vi "Init DH20vi.vi"(8 "error in (no error)":errorcluster, 11 "Grove Temperature Humidity Sensor DH20 in":refnum<class "Grove Temperature Humidity Sensor DH20.lvclass">) -> (0 "error out":errorcluster, 3 "6Grove Temperature Humidity Sensor DH20 out":refnum<class "Grove Temperature Humidity Sensor DH20.lvclass">)   [LabVIEW 2020, in "CTI-Peripheral.lvlib" / "Grove Temperature Humidity Sensor DH20.lvclass"]
uses:
  Grove Temperature Humidity Sensor DH20.lvclass
  Grove Temperature Humidity Sensor DH20.lvclass/Grove Temperature Humidity Sensor DH20.ctl
  CTI/I2C Connection/I2C Connection.lvclass/I2C Connection.ctl
  CTI/Session/I2C Write Data.vi
  CTI/Session/I2C Read Data.vi
  CTI/I2C Connection/I2C Connection.lvclass
panel:
  out "TimedOut":bool
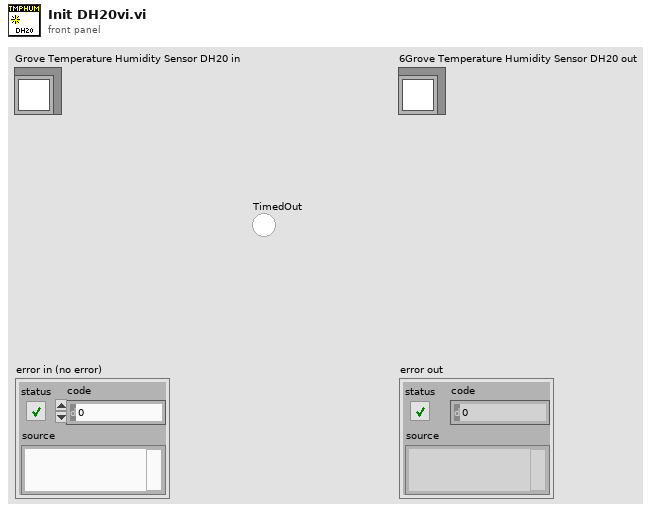
[diagram p1: front panel]
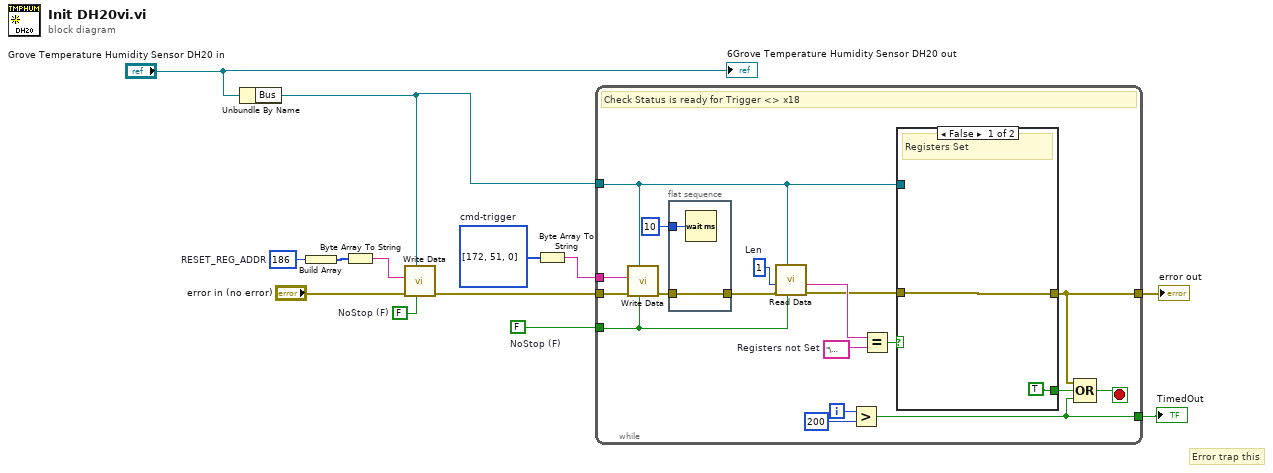
[diagram p0: block diagram]
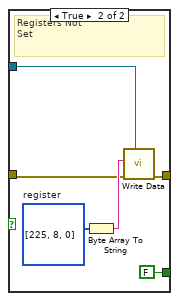
[diagram p2: hidden frame]
diagram:
  w2 = FALSE  # NoStop (F)
  w7 = FALSE  # NoStop (F)
  w9 = u8[] [172, 51, 0]  # cmd-trigger
  w12 = u8 186  # RESET_REG_ADDR
  # "Error trap this"
  n1 = Unbundle By Name("Grove Temperature Humidity Sensor DH20 in") -> ("Bus"=w3:refnum<class "I2C Connection.lvclass">)
  n2 = Build Array(w12) -> (w11:u8[])
  n3 = Byte Array To String(unsigned byte array=w11) -> (string=w6:string)
  n4 = call "Write Data.vi"("NoStop (F)"=w7, "I2C Connection"=w3, "error in (no error)"="error in (no error)", "Data"=w6) -> ("error out"=w4:errorcluster)  [unwired: 7 in]
  n5 = Byte Array To String(unsigned byte array=w9) -> (string=w8:string)
  n6 = while {
    tunnel: w4 -> [w23]
    tunnel: w8 -> [w22]
    tunnel: [w25] -> w1
    tunnel: [w27] -> w10
    tunnel: w3 -> [w14]
    tunnel: w2 -> [w18]
    i -> [w30]
    stop <- w28 stop-if-true
    w19 = u8 1  # Len
    w31 = "\u0018"  # Registers not Set
    # "Check Status is ready for Trigger <> x18"
    n7 = call "Write Data.vi"("NoStop (F)"=w18, "I2C Connection"=w14, "error in (no error)"=w23, "Data"=w22) -> ("error out"=w21:errorcluster)  [unwired: 7 in]
    n8 = flat-sequence {
      tunnel: w21 -> [w32]
      tunnel: u32 10 ("milliseconds to wait") -> [w33]
      tunnel: [w32] -> w17
      frame #0 {
        n9 = Wait (ms)(milliseconds to wait=w33) -> ()  [unwired: 1 out]
      }
    }
    n10 = call "Read Data.vi"("NoStop (F)"=w18, "I2C Connection"=w14, "error in (no error)"=w17, "Len"=w19) -> ("error out"=w15:errorcluster, "Data"=w16:string)  [unwired: 6 in]
    n11 = Greater?(x=w30, y=200) -> (0:w27:bool)
    n12 = Equal?(x=w16, y=w31) -> (x = y?=w26:bool)
    n13 = case shown="False" w26 {
      tunnel: w15 -> [w35 w38]
      tunnel: [w35 w37] -> w25
      tunnel: [TRUE FALSE] -> w24
      tunnel: w14 -> [_ w36]
      frame False {
        # "Registers Set"
      }
      frame True {
        w40 = u8[] [225, 8, 0]  # register
        # "Registers Not\nSet"
        n14 = Byte Array To String(unsigned byte array=w40) -> (string=w39:string)
        n15 = call "Write Data.vi"("I2C Connection"=w36, "error in (no error)"=w38, "Data"=w39) -> ("error out"=w37:errorcluster)  [unwired: 8 in]
      }
    }
    n16 = Compound Arithmetic op=OR(w25, w24, w27) -> (w28:bool)
  }
  "error out" <- w1
  "TimedOut" <- w10
  "6Grove Temperature Humidity Sensor DH20 out" <- "Grove Temperature Humidity Sensor DH20 in"
